vi "q3 boolean logic.vi"() -> ()   [LabVIEW 2025]
panel:
  out "Y":bool
  in  "D":bool
  in  "C":bool
  in  "B":bool
  in  "A":bool
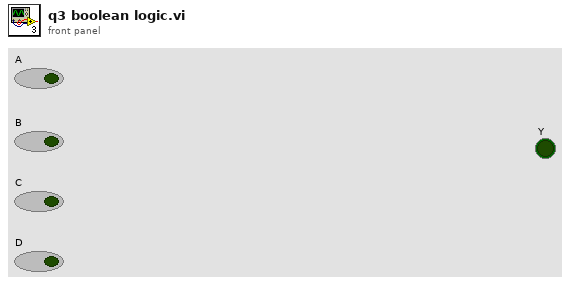
[diagram p1: front panel]
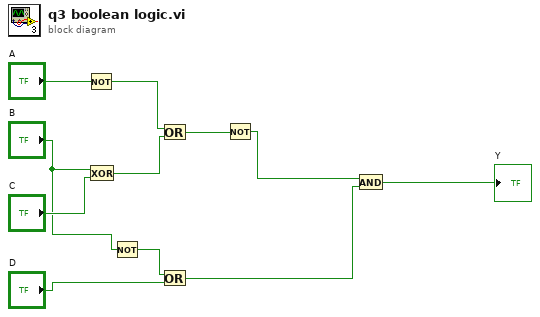
[diagram p0: block diagram]
diagram:
  n1 = Not(x="A") -> (.not. x?=w9:bool)
  n2 = Exclusive Or(1:"C", 2:"B") -> (0:w8:bool)
  n3 = Not(x="B") -> (.not. x?=w5:bool)
  n4 = Or(x=w9, y=w8) -> (x .or. y?=w7:bool)
  n5 = Or(x=w5, y="D") -> (x .or. y?=w2:bool)
  n6 = Not(x=w7) -> (.not. x?=w3:bool)
  n7 = And(x=w3, y=w2) -> (x .and. y?=→"Y":bool)
